vi "DCPower_CurrentLimitConfiguration.vi"(8 "error in (no error)":errorcluster, 9 "current limit":dbl, 10 "Active Channel Numbers String":string, 11 "IVI Refnum in":refnum<k15>) -> (0 "error out":errorcluster, 3 "IVI Refnum out":refnum<k15>)   [LabVIEW 2019]
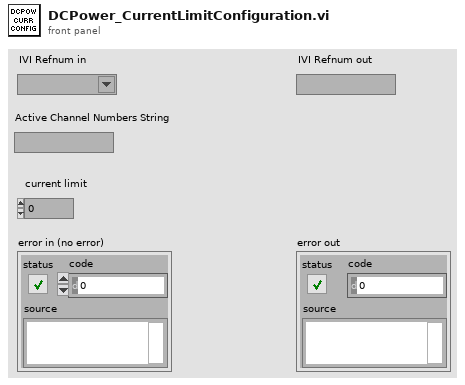
[diagram p1: front panel]
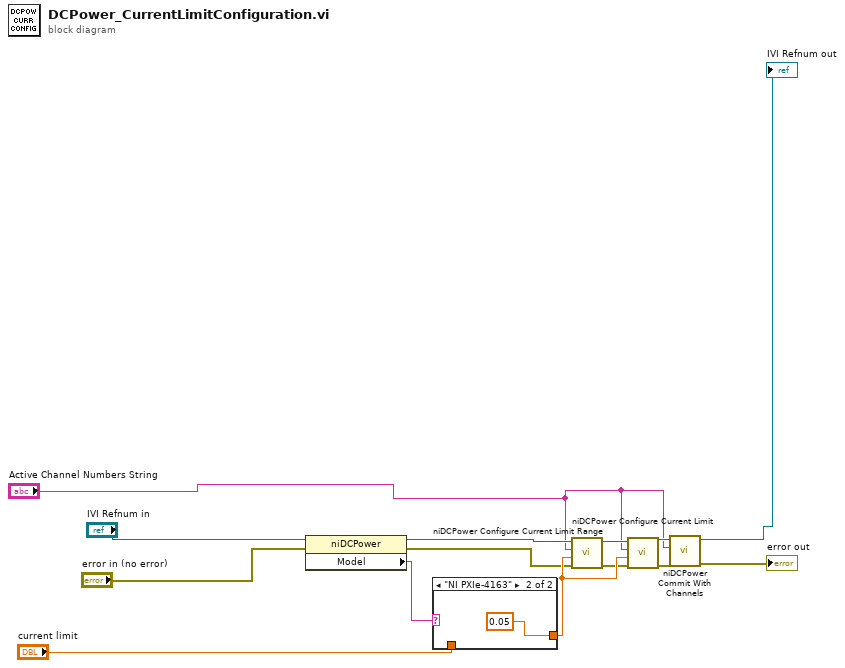
[diagram p0: block diagram]
diagram:
  n1 = property class="niDCPower"(reference="IVI Refnum in", error in="error in (no error)") -> (reference out=w4:refnum<k15>, error out=w5:errorcluster, "Model"=w6:string)
  n2 = case shown="\"NI PXIe-4163\"" w6 {
    tunnel: "current limit" -> [w15 _]
    tunnel: [w15 0.05 ("current limit")] -> w7
    frame Default {
    }
    frame "NI PXIe-4163" {
    }
  }
  n3 = call <instrlib>:"niDCPower Configure Current Limit Range.vi"("error in (no error)"=w5, "current limit range"=w7, "channel name"="Active Channel Numbers String", "instrument handle"=w4) -> ("error out"=w2:errorcluster, "instrument handle out"=w3:refnum<k15>)  [unwired: 6 in]
  n4 = call <instrlib>:"niDCPower Configure Current Limit.vi"("error in (no error)"=w2, "current limit"=w7, "channel name"="Active Channel Numbers String", "instrument handle"=w3) -> ("error out"=w9:errorcluster, "instrument handle out"=w8:refnum<k15>)  [unwired: 6 in]
  n5 = call <instrlib>:"niDCPower Commit With Channels.vi"("error in (no error)"=w9, "channel name"="Active Channel Numbers String", "instrument handle"=w8) -> ("error out"=→"error out":errorcluster, "instrument handle out"=→"IVI Refnum out":refnum<k15>)  [unwired: 7 in]
